vi "_DRIVER_SHARED_INI_ReadINICharacteristics.vi"(8 "error in":errorcluster, 10 "Driver to Sel":string, 11 "Path of \"_HW-Configuration_.ini\"":path=path "C:/UG-WORK/_DRIVER_/LV2020/NI9205/_HW-Configuration_.ini") -> (0 "error out":errorcluster, 3 "INPUT Values":T1[](array[typedef]))   [LabVIEW 2020]
doc: "This VI checks if the \"Driver to Sel\" is found in \"_HW-Configuration_.ini\" by its path. If found return an array of \"INPUTS - SUBSECTION\" need to initialize the driver. If the \"Driver to Sel\" is not found returns an error."
uses:
  TYPEDEF/_DRIVER_SHARED_TYPEDEF_StringControlVaviables.ctl
  TYPEDEF/_DRIVER_SHARED_TYPEDEF_INI-Method.ctl
  <vilib>/Utility/error.llb/Error Cluster From Error Code.vi
  <vilib>/ErrorRing/Error Ring.xnode
  <vilib>/Utility/config.llb/NI_LVConfig.lvlib
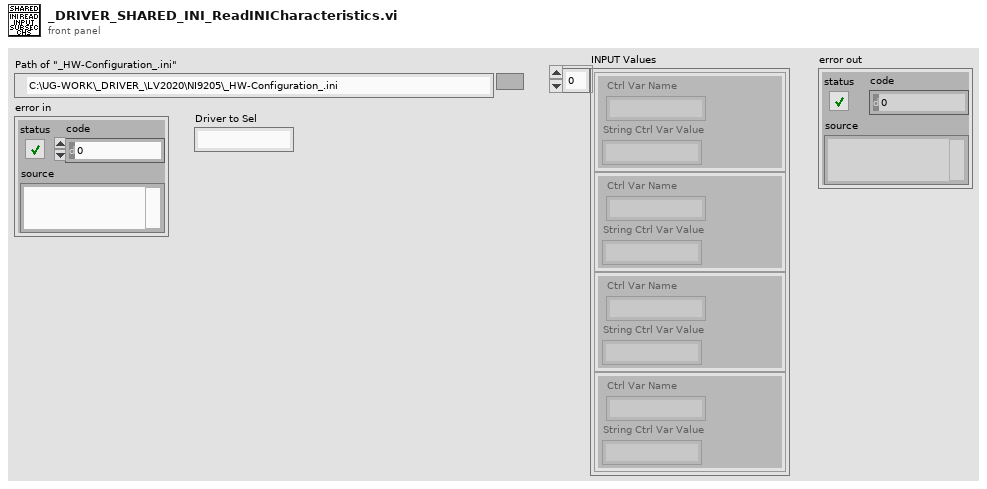
[diagram p1: front panel]
types:
  T1 = typedef "_DRIVER_SHARED_TYPEDEF_StringControlVaviables.ctl" = cluster{"Ctrl Var Name":string, "String Ctrl Var Value":string}
  T2 = enum16{"OpenFile", "CheckBoardbyType", "Verify If Inputs", "Read Controls", "Close File"}
  T3 = typedef "_DRIVER_SHARED_TYPEDEF_INI-Method.ctl" = enum16{"OPEN/CREATE", "READ", "WRITE", "CLOSE", "NO_OP"}
  T4 = typedef "NI_LVConfig.lvlib/Config Data RefNum.ctl" = refnum<k1>
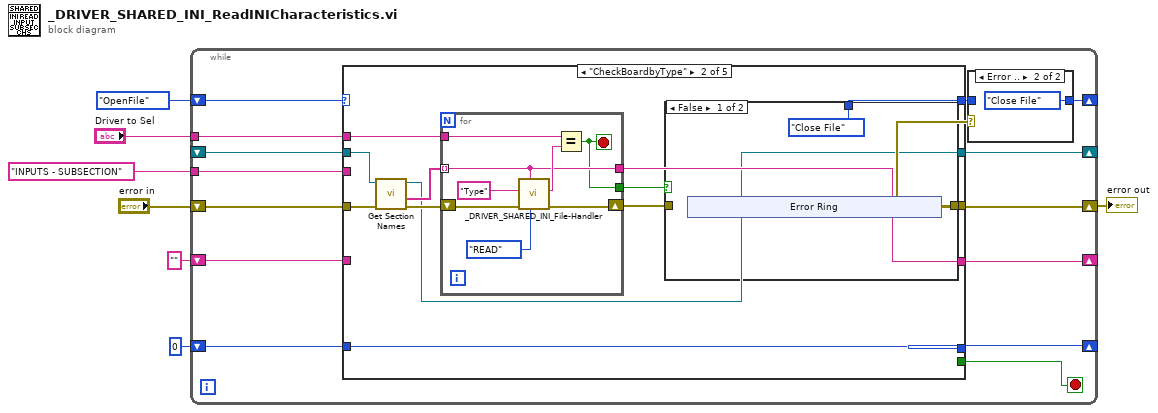
[diagram p0: block diagram]
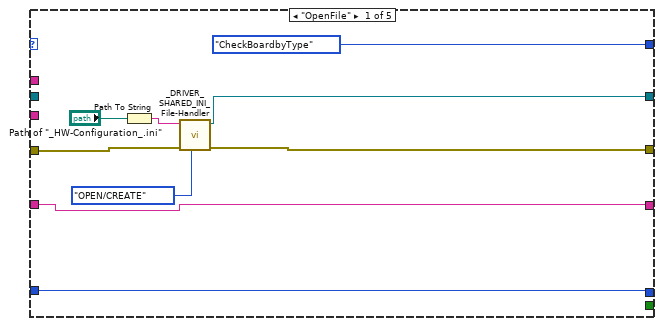
[diagram p3: hidden frame]
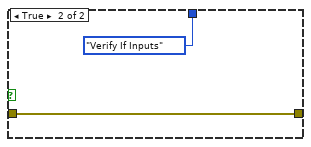
[diagram p4: hidden frame]
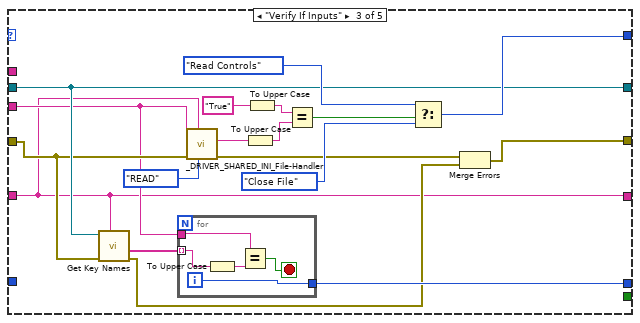
[diagram p5: hidden frame]
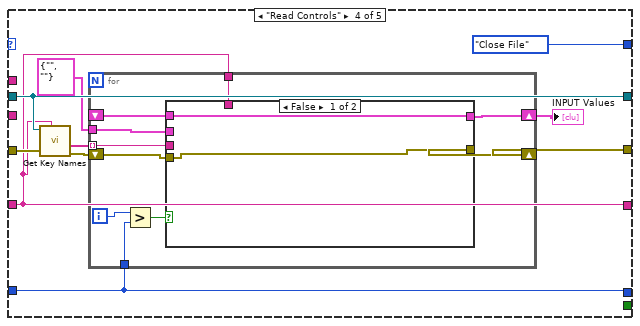
[diagram p6: hidden frame]
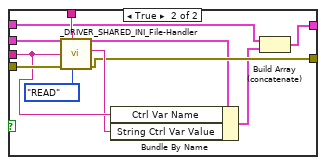
[diagram p7: hidden frame]
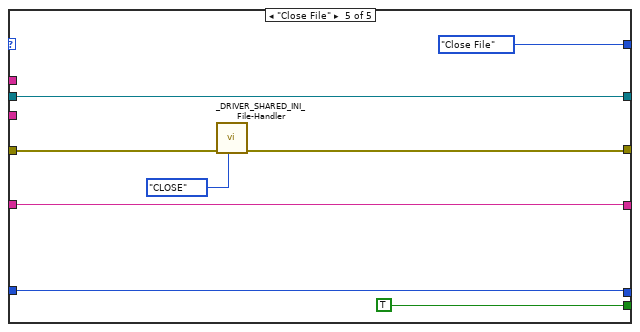
[diagram p8: hidden frame]
diagram:
  n1 = while {
    shift-right: [w17] -> w5
    shift-left: "error in" -> [w20]
    shift-right: [w19] -> _
    shift-left: T2."OpenFile" -> [w21]
    shift-right: [w16] -> _
    shift-left: _ -> [w15]
    tunnel: "Driver to Sel" -> [w14]
    shift-right: [w13] -> _
    shift-left: "" ("String") -> [w12]
    tunnel: "INPUTS - SUBSECTION" ("Path File") -> [w11]
    shift-right: [w10] -> _
    shift-left: 0 -> [w9]
    stop <- w8 stop-if-true
    n2 = case shown="\"CheckBoardbyType\"" w21 {
      tunnel: [w27 w33 w64 w89 w118] -> w17
      tunnel: w20 -> [w29 w43 w69 w94 w119]
      tunnel: [T2."CheckBoardbyType" w34 w71 T2."Close File" T2."Close File"] -> w18
      tunnel: [w26 w38 w70 w93 w124] -> w16
      tunnel: w15 -> [_ w44 w70 w93 w124]
      tunnel: w14 -> [_ w40 _ _ _]
      tunnel: [w25 w39 w62 w87 w123] -> w13
      tunnel: w12 -> [w25 _ w62 w87 w123]
      tunnel: w11 -> [_ _ w67 _ _]
      tunnel: [w24 w37 w66 w91 w122] -> w10
      tunnel: w9 -> [w24 w37 _ w91 w122]
      tunnel: [_ _ _ _ TRUE] -> w8
      frame "OpenFile" {
        n3 = Path To String(path="Path of \"_HW-Configuration_.ini\"") -> (string=w30:string)
        n4 = call "_DRIVER_SHARED_INI_File-Handler.vi"("INI-FileMethod"=_DRIVER_SHARED_TYPEDEF_INI-Method."OPEN/CREATE", "error in (no error)"=w29, "Path File"=w30) -> ("error out"=w27:errorcluster, "refnum out"=w26:T4)  [unwired: 6 in, 1 out]
      }
      frame "CheckBoardbyType" {
        n5 = call <vilib>:"Get Section Names.vi"("error in (no error)"=w43, "refnum"=w44) -> ("error out"=w41:errorcluster, "section names"=w42:string[], "refnum out"=w38:T4)  [unwired: 7 in]
        n6 = for {
          tunnel: w42 -> [w55] mode=indexing
          shift-right: [w58] -> w35
          shift-left: w41 -> [w59]
          tunnel: w40 -> [w56]
          tunnel: [w55] -> w39
          tunnel: [w54] -> w36
          stop <- w54 stop-if-true
          n7 = call "_DRIVER_SHARED_INI_File-Handler.vi"("INI-FileMethod"=_DRIVER_SHARED_TYPEDEF_INI-Method."READ", "section IN"=w55, "error in (no error)"=w59, "key IN"="Type") -> ("error out"=w58:errorcluster, "value Read"=w57:string)  [unwired: 5 in, 1 out]
          n8 = Equal?(x=w56, y=w57) -> (x = y?=w54:bool)
        }
        n9 = case shown="False" w36 {
          tunnel: w35 -> [_ w52]
          tunnel: [T2."Close File" T2."Verify If Inputs"] -> w34
          tunnel: [w45 w52] -> w33
          frame False {
            n10 = xnode "Error Ring"() -> ("error out"=w45:errorcluster)
          }
          frame True {
          }
        }
      }
      frame "Verify If Inputs" {
        n11 = call <vilib>:"Get Key Names.vi"("section"=w62, "error in (no error)"=w69, "refnum"=w70) -> ("error out"=w63:errorcluster, "key names"=w68:string[])  [unwired: 5 in, 2 out]
        n12 = for {
          tunnel: w68 -> [w84] mode=indexing
          tunnel: w67 -> [w82]
          tunnel: [w80] -> w66
          i -> [w80]
          stop <- w81 stop-if-true
          n13 = To Upper Case(1:w84) -> (0:w83:string)
          n14 = Equal?(x=w82, y=w83) -> (x = y?=w81:bool)
        }
        n15 = call "_DRIVER_SHARED_INI_File-Handler.vi"("INI-FileMethod"=_DRIVER_SHARED_TYPEDEF_INI-Method."READ", "section IN"=w62, "error in (no error)"=w69, "key IN"=w67) -> ("error out"=w65:errorcluster, "value Read"=w75:string)  [unwired: 5 in, 1 out]
        n16 = To Upper Case(1:w75) -> (0:w76:string)
        n17 = To Upper Case(1:"True" ("string")) -> (0:w77:string)
        n18 = Equal?(x=w77, y=w76) -> (x = y?=w74:bool)
        n19 = Select(t=T2."Read Controls", s=w74, f=T2."Close File") -> (s? t:f=w71:T2)
        n20 = Merge Errors(w65, w63) -> (w64:errorcluster)
      }
      frame "Read Controls" {
        n21 = call <vilib>:"Get Key Names.vi"("section"=w87, "error in (no error)"=w94, "refnum"=w93) -> ("error out"=w90:errorcluster, "key names"=w92:string[])  [unwired: 5 in, 2 out]
        n22 = for {
          tunnel: w92 -> [w101] mode=indexing
          tunnel: w91 -> [w103]
          tunnel: w87 -> [w100]
          shift-right: [w98] -> w89
          shift-left: w90 -> [w99]
          tunnel: T1 {"Ctrl Var Name"="", "String Ctrl Var Value"=""} ("String Control Variables") -> [w97]
          shift-right: [w96] -> w85
          shift-left: _ -> [w95]
          i -> [w104]
          n23 = Greater?(x=w104, y=w103) -> (0:w102:bool)
          n24 = case shown="False" w102 {
            tunnel: w101 -> [_ w113]
            tunnel: w100 -> [_ w115]
            tunnel: w99 -> [w106 w114]
            tunnel: w97 -> [_ w108]
            tunnel: [w105 w109] -> w96
            tunnel: [w106 w111] -> w98
            tunnel: w95 -> [w105 w107]
            frame False {
            }
            frame True {
              n25 = call "_DRIVER_SHARED_INI_File-Handler.vi"("INI-FileMethod"=_DRIVER_SHARED_TYPEDEF_INI-Method."READ", "section IN"=w115, "error in (no error)"=w114, "key IN"=w113) -> ("error out"=w111:errorcluster, "value Read"=w112:string)  [unwired: 5 in, 1 out]
              n26 = Bundle By Name(cluster=w108, "Ctrl Var Name"=w113, "String Ctrl Var Value"=w112) -> (w110:T1)
              n27 = Build Array (concatenate)(w107, w110) -> (w109:T1[])
            }
          }
        }
        "INPUT Values" <- w85
      }
      frame "Close File" {
        n28 = call "_DRIVER_SHARED_INI_File-Handler.vi"("INI-FileMethod"=_DRIVER_SHARED_TYPEDEF_INI-Method."CLOSE", "error in (no error)"=w119) -> ("error out"=w118:errorcluster)  [unwired: 7 in, 2 out]
      }
    }
    n29 = case shown="Error .." w17 {
      tunnel: [w22 T2."Close File"] -> w19
      tunnel: w18 -> [w22 _]
      frame No Error {
      }
      frame Error {
      }
    }
  }
  "error out" <- w5
